vi "Return Variant.vi"(5 "Enum":T1(ring)) -> (4 "Numeric Measurement":variant, 8 "Report Text":string, 15 "error out":errorcluster)   [LabVIEW 2014]
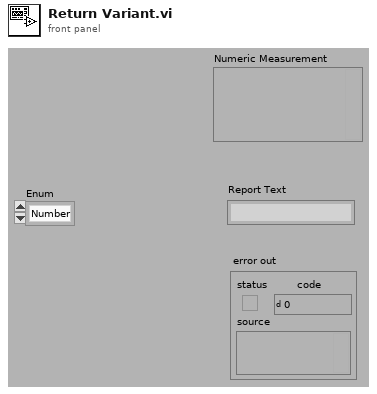
[diagram p1: front panel]
types:
  T1 = enum16{"Number", "ArrayOfNumbers", "String", "ArrayOfStrings"}
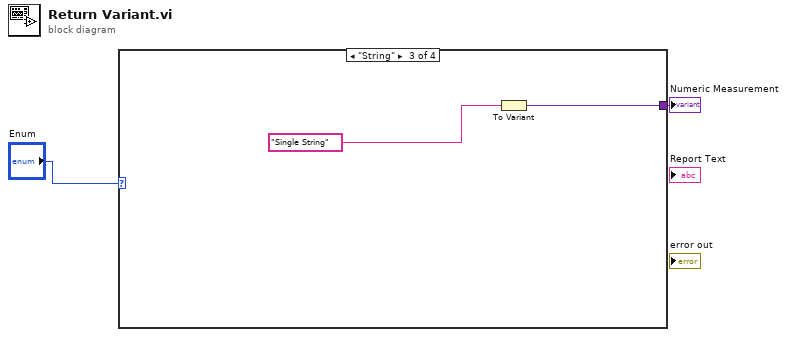
[diagram p0: block diagram]
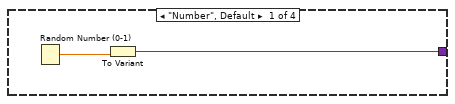
[diagram p2: hidden frame]
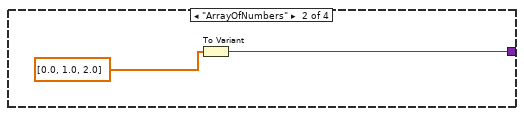
[diagram p3: hidden frame]
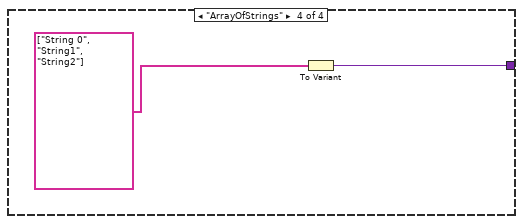
[diagram p4: hidden frame]
diagram:
  n1 = case shown="\"String\"" "Enum" {
    tunnel: [w3 w6 w8 w9] -> w1
    frame "Number", Default {
      n2 = Random Number (0-1)() -> (number: 0 to 1=w4:dbl)
      n3 = To Variant(anything=w4) -> (Variant=w3:variant)
    }
    frame "ArrayOfNumbers" {
      n4 = To Variant(anything=dbl[] [0.0, 1.0, 2.0]) -> (Variant=w6:variant)
    }
    frame "String" {
      n5 = To Variant(anything="Single String" ("Report Text")) -> (Variant=w8:variant)
    }
    frame "ArrayOfStrings" {
      n6 = To Variant(anything=string[] ["String 0", "String1", "String2"]) -> (Variant=w9:variant)
    }
  }
  "Numeric Measurement" <- w1
